vi "GetSSLLibraryPath.vi"(8 "error in (no error)":errorcluster) -> (0 "error out":errorcluster, 1 "CA-bundle.crt":string, 2 "NIssleay library path":path, 3 "NIlibeay library pat":path)   [LabVIEW 2015, in "AWS_IoT.lvlib"]
uses:
  <vilib>/Utility/sysdir.llb/System Directory Type.ctl
  AWS_IoT.lvlib
panel:
  out "CA-bundle.crt":path
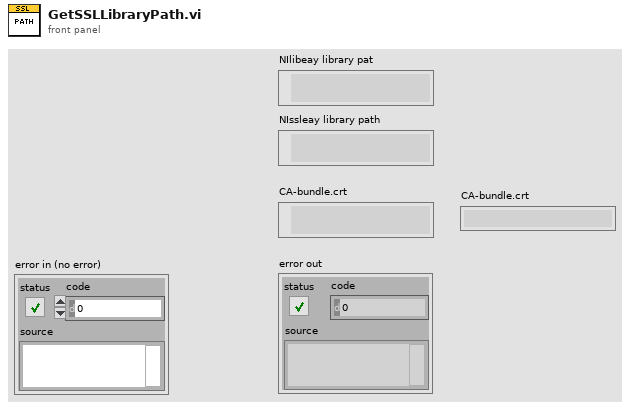
[diagram p1: front panel]
types:
  T1 = typedef "System Directory Type.ctl" = i32
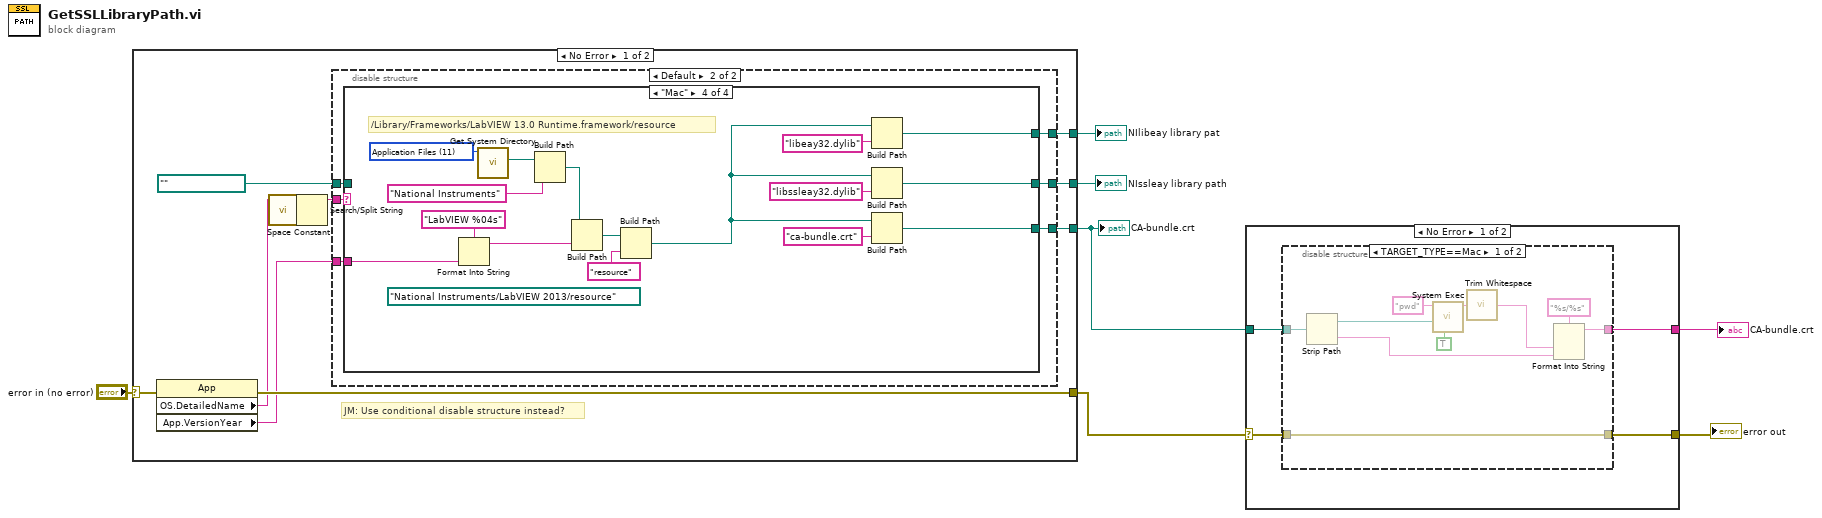
[diagram p0: block diagram]
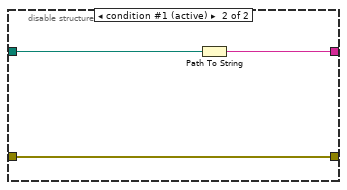
[diagram p2: hidden frame]
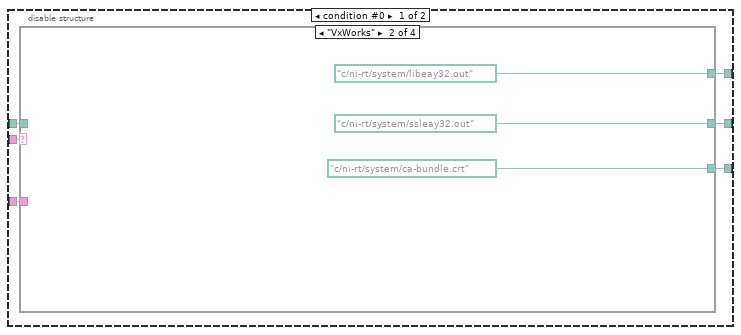
[diagram p4: hidden frame]
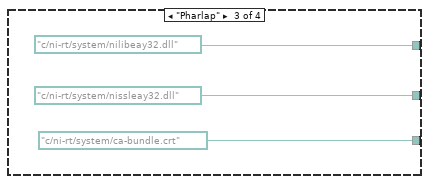
[diagram p6: hidden frame]
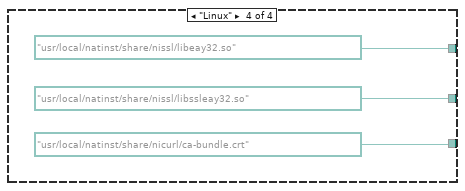
[diagram p7: hidden frame]
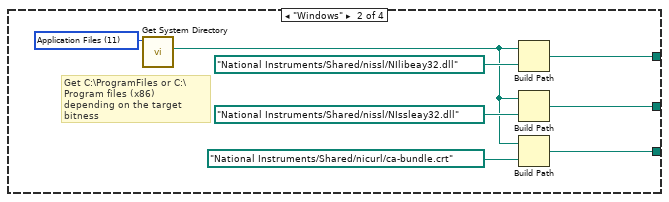
[diagram p9: hidden frame]
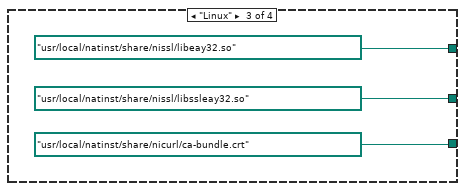
[diagram p10: hidden frame]
diagram:
  n1 = case shown="No Error" "error in (no error)" {
    selector: "error in (no error)" -> [w15 w68]
    tunnel: [w17 _] -> w7
    tunnel: [w14 w68] -> w3
    tunnel: [w10 _] -> w4
    tunnel: [w9 _] -> w6
    frame No Error {
      # "JM: Use conditional disable structure instead?"
      n2 = property class="App"(error in=w15) -> (error out=w14:errorcluster, "OS.DetailedName"=w13:string, "App.VersionYear"=w8:string)  [unwired: 1 in, 1 out]
      n3 = call <vilib>:"Space Constant.vi"() -> ("String"=w12:string)
      n4 = Search/Split String(string=w13, search string/char (-)=w12) -> (substring before match=w11:string)  [unwired: 1 in, 2 out]
      n5 = disable-structure shown="Default" {
        disable-tunnel: [w23 w39] -> w17
        disable-tunnel: path "" ("SSL library path") -> [w22 w38]
        disable-tunnel: w11 -> [w21 w37]
        disable-tunnel: [w20 w36] -> w10
        disable-tunnel: [w19 w35] -> w9
        disable-tunnel: w8 -> [w18 w34]
        frame condition #0 {
          n6 = case shown="\"VxWorks\"" w21 {
            tunnel: [w24 path "c:/ni-rt/system/ssleay32.out" ("SSL library path") path "c:/ni-rt/system/nissleay32.dll" ("SSL library path") path "/usr/local/natinst/share/nissl/libssleay32.so" ("SSL library path")] -> w23
            tunnel: w22 -> [w24 _ _ _]
            tunnel: [w24 path "c:/ni-rt/system/ca-bundle.crt" ("SSL library path") path "c:/ni-rt/system/ca-bundle.crt" ("SSL library path") path "/usr/local/natinst/share/nicurl/ca-bundle.crt" ("SSL library path")] -> w20
            tunnel: [w24 path "c:/ni-rt/system/libeay32.out" ("SSL library path") path "c:/ni-rt/system/nilibeay32.dll" ("SSL library path") path "/usr/local/natinst/share/nissl/libeay32.so" ("SSL library path")] -> w19
            tunnel: w18 -> [_ _ _ _]
            frame "False", Default {
            }
            frame "VxWorks" {
            }
            frame "Pharlap" {
            }
            frame "Linux" {
            }
          }
        }
        frame condition #1 (active) {
          n7 = case shown="\"Mac\"" w37 {
            tunnel: [w40 w45 path "/usr/local/natinst/share/nissl/libssleay32.so" ("SSL library path") w64] -> w39
            tunnel: w38 -> [w40 _ _ _]
            tunnel: [w40 w44 path "/usr/local/natinst/share/nicurl/ca-bundle.crt" ("SSL library path") w54] -> w36
            tunnel: [w40 w47 path "/usr/local/natinst/share/nissl/libeay32.so" ("SSL library path") w65] -> w35
            tunnel: w34 -> [_ _ _ w60]
            frame "False", Default {
            }
            frame "Windows" {
              w42 = T1 11 items=["User Home"=0, "User Desktop"=1, "User Documents"=2, "User Application Data"=3, "User Preferences"=4, "User Temporary"=5, "Public Documents"=6, "Public Application Data"=7, "Public Preferences"=8, "Public Cache"=13, "System Core Libraries"=9, "System Installed Libraries"=10, "Application Files"=11, "Boot Volume Root"=12] ("system directory type")
              # "Get C:\\ProgramFiles or C:\\Program files (x86) depending on the target bitness"
              n8 = call <vilib>:"Get System Directory.vi"("system directory type"=w42) -> ("system directory"=w41:path)  [unwired: 10 in]
              n9 = Build Path(base path=w41, name or relative path=path "National Instruments/Shared/nissl/NIlibeay32.dll" ("SSL library path")) -> (appended path=w47:path)
              n10 = Build Path(base path=w41, name or relative path=path "National Instruments/Shared/nissl/NIssleay32.dll" ("SSL library path")) -> (appended path=w45:path)
              n11 = Build Path(base path=w41, name or relative path=path "National Instruments/Shared/nicurl/ca-bundle.crt" ("CAfile")) -> (appended path=w44:path)
            }
            frame "Linux" {
            }
            frame "Mac" {
              (unwired) path "National Instruments/LabVIEW 2013/resource"
              w67 = T1 11 items=["User Home"=0, "User Desktop"=1, "User Documents"=2, "User Application Data"=3, "User Preferences"=4, "User Temporary"=5, "Public Documents"=6, "Public Application Data"=7, "Public Preferences"=8, "Public Cache"=13, "System Core Libraries"=9, "System Installed Libraries"=10, "Application Files"=11, "Boot Volume Root"=12] ("system directory type")
              # "/Library/Frameworks/LabVIEW 13.0 Runtime.framework/resource"
              n12 = Format Into String(format string="LabVIEW %04s" ("command line"), w60) -> (resulting string=w58:string)  [unwired: 2 in, 1 out]
              n13 = call <vilib>:"Get System Directory.vi"("system directory type"=w67) -> ("system directory"=w66:path)  [unwired: 10 in]
              n14 = Build Path(base path=w66, name or relative path="National Instruments" ("command line")) -> (appended path=w55:path)
              n15 = Build Path(base path=w55, name or relative path=w58) -> (appended path=w57:path)
              n16 = Build Path(base path=w57, name or relative path="resource" ("command line")) -> (appended path=w53:path)
              n17 = Build Path(base path=w53, name or relative path="libeay32.dylib") -> (appended path=w65:path)
              n18 = Build Path(base path=w53, name or relative path="libssleay32.dylib") -> (appended path=w64:path)
              n19 = Build Path(base path=w53, name or relative path="ca-bundle.crt") -> (appended path=w54:path)
            }
          }
        }
      }
    }
    frame Error {
    }
  }
  "NIssleay library path" <- w7
  "CA-bundle.crt" <- w4
  "NIlibeay library pat" <- w6
  n20 = case shown="No Error" w3 {
    selector: w3 -> [w72 w86]
    tunnel: [w70 w86] -> w2
    tunnel: [w69 _] -> w1
    tunnel: w4 -> [w71 _]
    frame No Error {
      n21 = disable-structure shown="TARGET_TYPE==Mac" {
        disable-tunnel: w72 -> [w78 w83]
        disable-tunnel: w71 -> [w77 w85]
        disable-tunnel: [w73 w84] -> w69
        disable-tunnel: [w78 w83] -> w70
        frame condition #0 {
          n22 = Strip Path(path=w77) -> (stripped path=w76:path, name=w74:string)
          n23 = call <vilib>:"System Exec.vi"("run minimized? (F)"=TRUE, "working directory"=w76, "command line"="pwd") -> ("standard output"=w79:string)  [unwired: 5 in, 3 out]
          n24 = call <vilib>:"Trim Whitespace.vi"("string"=w79) -> ("trimmed string"=w75:string)  [unwired: 1 in]
          n25 = Format Into String(format string="%s/%s" ("name or relative path"), w75, w74) -> (resulting string=w73:string)  [unwired: 2 in, 1 out]
        }
        frame condition #1 (active) {
          n26 = Path To String(path=w85) -> (string=w84:string)
        }
      }
    }
    frame Error {
    }
  }
  "error out" <- w2
  "CA-bundle.crt" <- w1
